vi "Set Motor Gains.vi"(8 "error in (no error)":errorcluster, 10 "motor gains":T1, 11 "MF3 in":refnum<class "MF3.lvclass">) -> (0 "error out":errorcluster, 3 "MF3 out":refnum<class "MF3.lvclass">)   [LabVIEW 2013, in "MF3.lvclass"]
uses:
  MF3.lvclass
  MF3.lvclass/MF3.ctl
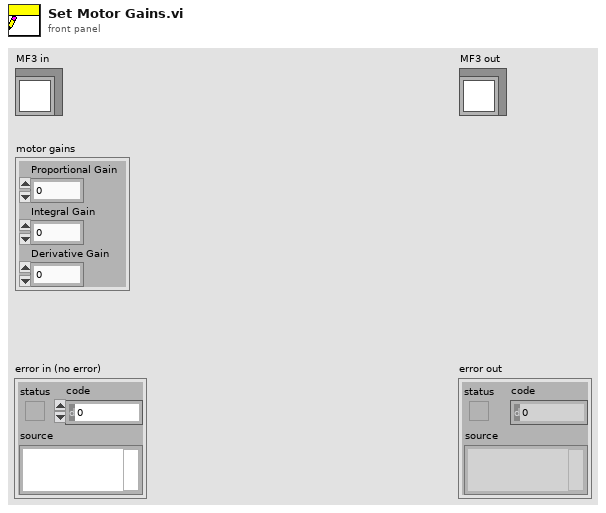
[diagram p1: front panel]
types:
  T1 = cluster{"Proportional Gain":i16, "Integral Gain":i16, "Derivative Gain":i16}
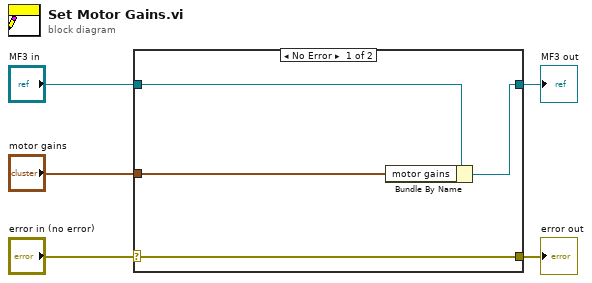
[diagram p0: block diagram]
diagram:
  n1 = case shown="No Error" "error in (no error)" {
    selector: "error in (no error)" -> [w9 w10]
    tunnel: [w9 w10] -> w4
    tunnel: [w7 w11] -> w2
    tunnel: "MF3 in" -> [w8 w11]
    tunnel: "motor gains" -> [w6 _]
    frame No Error {
      n2 = Bundle By Name(cluster=w8, "motor gains"=w6) -> (w7:refnum<class "MF3.lvclass">)
    }
    frame Error {
    }
  }
  "error out" <- w4
  "MF3 out" <- w2
